vi "Format Item Names.vi"(5 "Displayed Indices":i32[](array[numeric]), 7 "Abbreviate Names?":bool, 9 "Saved VI Data":T1[](array[typedef]), 11 "New VI Data":T1[](array[typedef])) -> (2 "Item Names":string[](array[string]))   [LabVIEW 2023, in "VI Properties Editor.lvlib"]
doc: "Formats the VI names into item names to be displayed in the main listbox, based on <B>Abbreviate Names?</B> and if modifications have been made."
uses:
  VI Properties Editor.lvlib
  CTLs/VI Data.ctl
  CTLs/VI Properties.ctl
  <vilib>/picture/picture.llb/imagedata.ctl
  CTLs/Control Properties.ctl
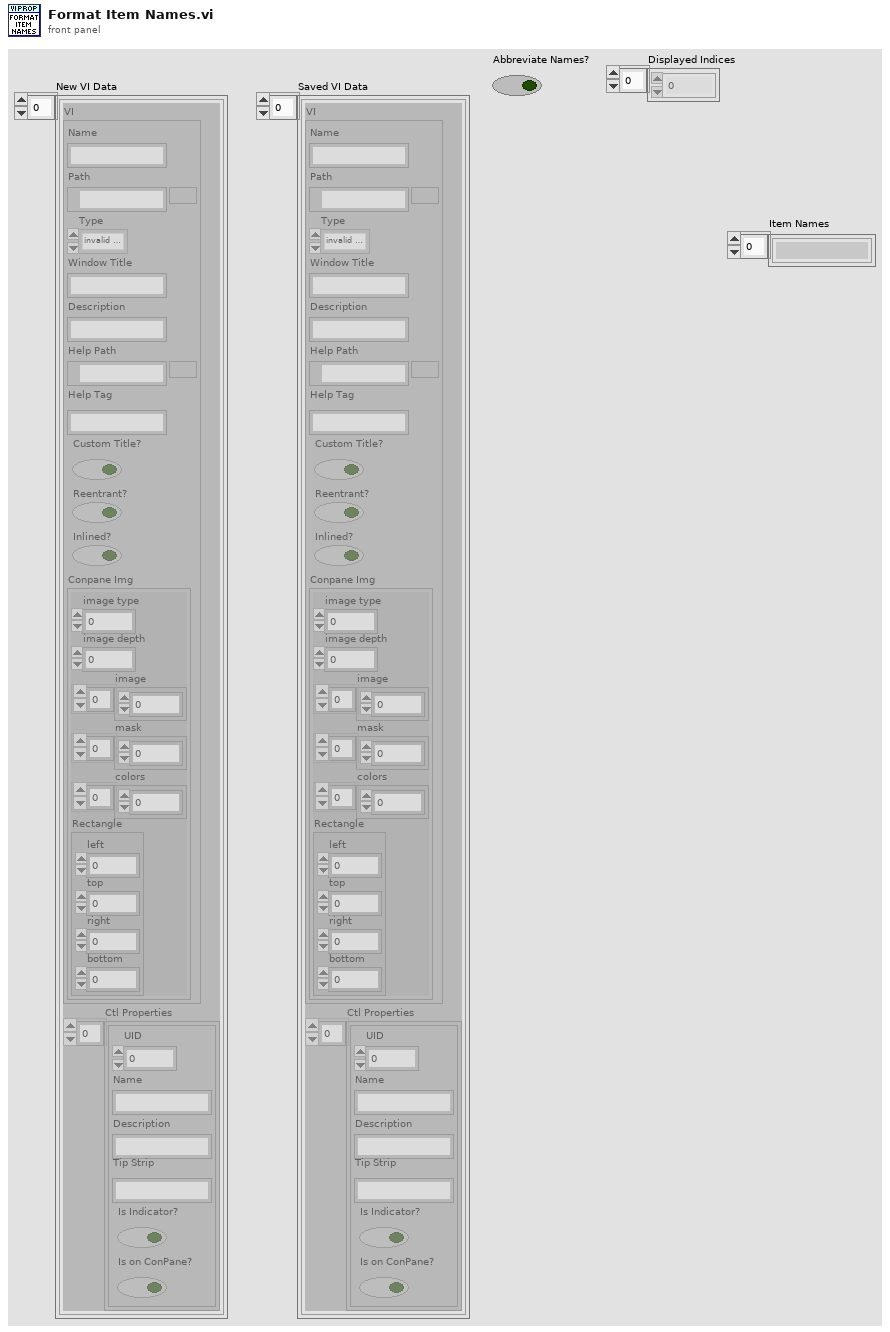
[diagram p1: front panel]
types:
  T1 = typedef "VI Properties Editor.lvlib/VI Data.ctl" = cluster{"VI":T2, "Ctl Properties":T4[]}
  T2 = typedef "VI Properties Editor.lvlib/VI Properties.ctl" = cluster{"Name":string, "Path":path, "Type":enum32{"invalid VI type", "Standard VI", "Control VI", "Global VI", "Polymorphic VI", "Configuration VI", "SubSystem", "Facade VI", "Method VI", "Statechart Diagram VI"}, "Window Title":string, "Description":string, "Help Path":path, "Help Tag":string, "Custom Title?":bool, "Reentrant?":bool, "Inlined?":bool, "Conpane Img":T3}
  T3 = typedef "imagedata.ctl" = cluster{"image type":i32, "image depth":i32, "image":u8[], "mask":u8[], "colors":u32[], "Rectangle":cluster{"left":i16, "top":i16, "right":i16, "bottom":i16}}
  T4 = typedef "VI Properties Editor.lvlib/Control Properties.ctl" = cluster{"UID":i32, "Name":string, "Description":string, "Tip Strip":string, "Is Indicator?":bool, "Is on ConPane?":bool}
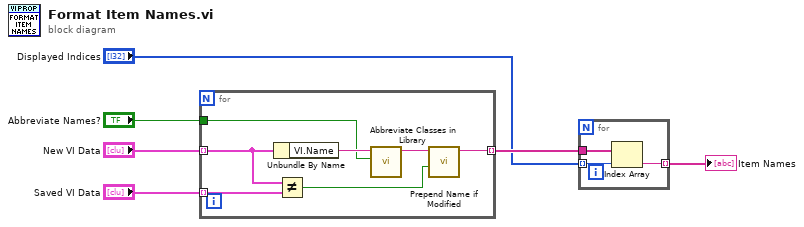
[diagram p0: block diagram]
diagram:
  n1 = for {
    tunnel: "Saved VI Data" -> [w13] mode=indexing
    tunnel: "New VI Data" -> [w12] mode=indexing
    tunnel: "Abbreviate Names?" -> [w10]
    tunnel: [w7] -> w3 mode=indexing
    n2 = Unbundle By Name(w12) -> ("VI.Name"=w11:string)
    n3 = Not Equal?(x=w12, y=w13) -> (x != y?=w8:bool)
    n4 = call "Abbreviate Classes in Library.vi"("Abbreviate Name?"=w10, "Name"=w11) -> ("Name out"=w9:string)  [unwired: 9 in]
    n5 = call "Prepend Name if Modified.vi"("Modified?"=w8, "VI Name"=w9) -> ("VI Name out"=w7:string)  [unwired: 9 in]
  }
  n6 = for {
    tunnel: w3 -> [w16]
    tunnel: "Displayed Indices" -> [w15] mode=indexing
    tunnel: [w14] -> w2 mode=indexing
    n7 = Index Array(array=w16, index=w15) -> (element=w14:string)
  }
  "Item Names" <- w2
